vi "asap_monitor.vi"() -> ()   [LabVIEW 2013]
uses:
  <vilib>/Analysis/Matrix/Datatypes/RealMatrix.ctl
  <vilib>/Platform/TimedLoop/XDataNode/timing_clust.ctl
  <vilib>/Platform/TimedLoop/XDataNode/nitl_modes.ctl
  <vilib>/Platform/TimedLoop/XDataNode/wakeup.ctl
  calibration/array_3d_double.ctl
  initialization/micron_globals.vi
  <vilib>/Platform/TimedLoop/XDataNode/XDataNode.xnode
  <vilib>/Platform/TimedLoop/XDataNode/XDNodeRunTimeDep.lvlib
  <vilib>/Analysis/Matrix/NI_Matrix.lvlib
panel:
  in  "To Trace Data":bool
  in  "stop":bool
  in  "Clear":bool
  out "Vector sum":dbl format="%#_4p"
  in  "Display":T1(ring)
  in  "Select":bool[](array[boolean])
  out "ASAP status":cluster{"Valid position":bool, "Message":string}
  out "Match error":sgl[](array[numeric]) format="%#.1f"
  out "Light triad error":dbl[](array[numeric]) format="%#.0f"
  out "Handle pose string":string
  out "Light position":sgl[](array[numeric]) format="%#.0f"
  out "Translation":dbl[](array[numeric]) format="%#.1f"
  out "Sum amplitudes":sgl[][](array[numeric]) format="%#.4f"
  out "Axis position":sgl[](array[numeric]) format="%#_4g"
  out "Total angle":dbl format="%#_4g"
  out "Relative angles":dbl[](array[numeric]) format="%#.1f"
  out "Ref pose":T2=[[1.0, 0.0, 0.0, 0.0], [0.0, 1.0, 0.0, 0.0], [0.0, 0.0, 1.0, 0.0], [0.0, 0.0, 0.0, 1.0]] format="%#.3f"
  in  "Absolute":bool
  out "Sensor views":cluster{sgl[], sgl[]}[](graph)
  in  "Demodulated signals bandwidth":sgl=3.0
  out "Handle pose":T2 format="%#.3f"
  in  "Light":i32
  out "Reference":dbl[][](array[numeric])
  in  "Set ref":bool
  out "Waveform Chart":dbl[][](graph)
  out "Signals":dbl[](array[numeric]) format="%#_4p"
  # "X"
  # "Z1"
  # "Y"
  # "Z2"
  # "Light"
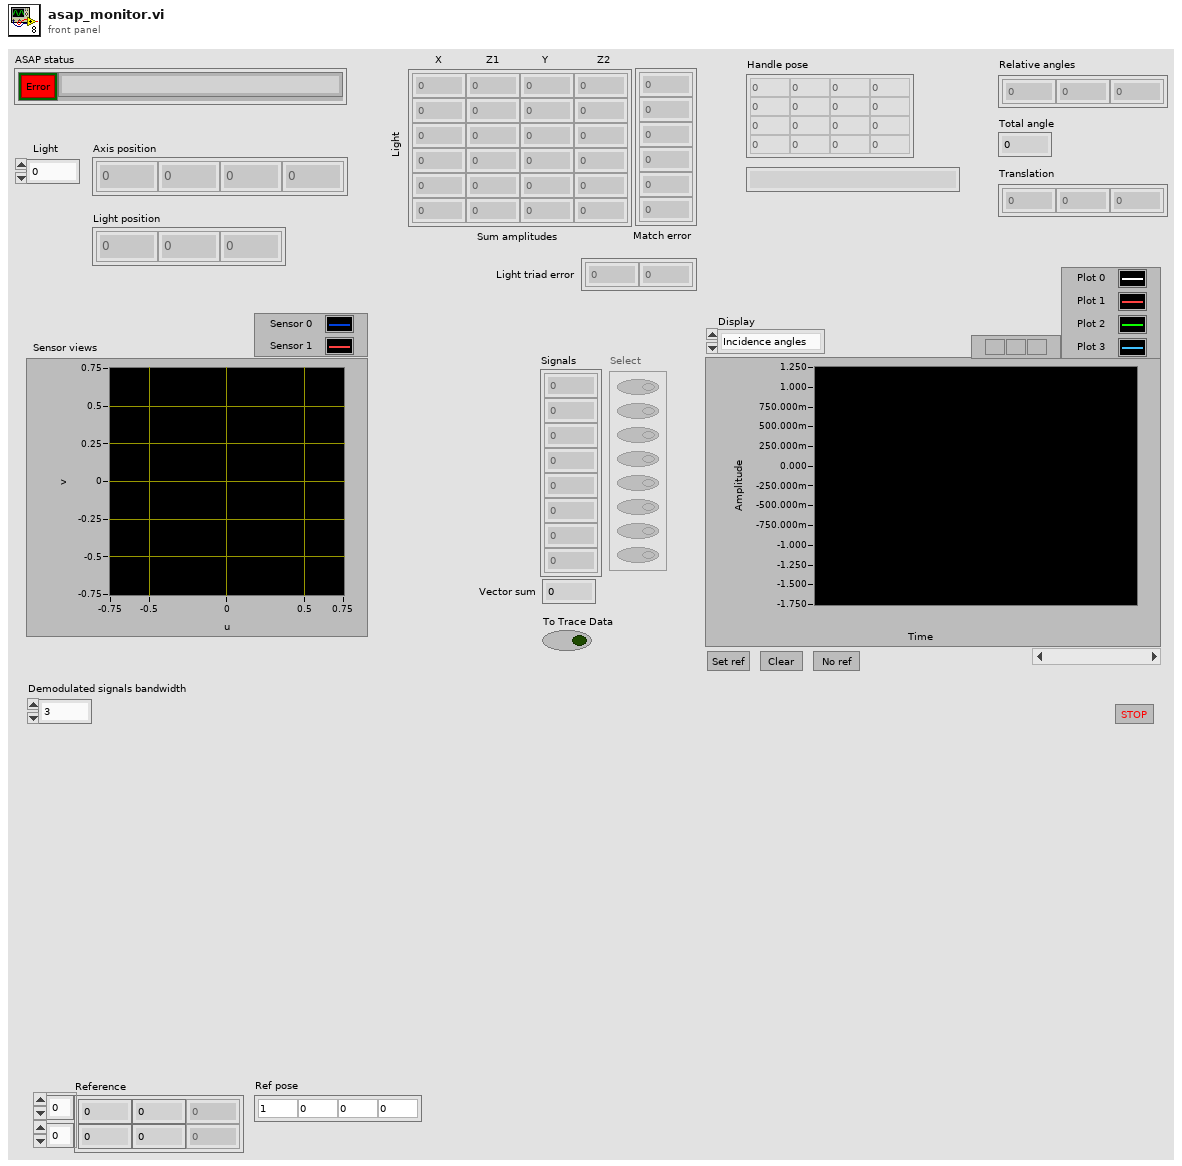
[diagram p1: front panel]
types:
  T1 = enum16{"Incidence angles", "Demod signals", "Sum amplitudes", "Difference signals", "Axis positions", "Light positions"}
  T2 = typedef "NI_Matrix.lvlib/RealMatrix.ctl" = dbl[][]
  T3 = typedef "configuration.ctl" = cluster{"Calibration data":T4, "Block size":i32, "Tasks":cluster{"Analog Input":refnum<k21>, "Counters":refnum<k21>[], "Digital out":refnum<k21>}, "Light enables":bool[]}
  T4 = typedef "asap_calibration.ctl" = cluster{"T1":T2, "K1":T2, "T2":T2, "K2":T2, "Sensor LUT":sgl[][][][]}
  T5 = typedef "micron_config.ctl" = cluster{"rt fifo":refnum<k33>, "Analog output task":refnum<k21>, "Analog output task 2":refnum<k21>, "Stimulus AO task":refnum<k21>, "Low-rate AIN task":refnum<k21>, "Pedal out task":refnum<k21>, "Pedal in task":refnum<k21>, "Loop timing source":string, "Relay out task":refnum<k21>, "Send UDP Conn":refnum<k16>, "Recv UDP Conn":refnum<k16>, "Host Addr":dbl, "I2C interface":T6, "trace_start notifier":refnum<notifier>, "trace_done notifier":refnum<notifier>, "ASAP FIFO":refnum<k33>}
  T6 = typedef "i2c_interface.ctl" = cluster{"FPGA VI Reference":T7}
  T7 = typedef "fpga_reference.ctl" = refnum<k20>
  T8 = typedef "XDNodeRunTimeDep.lvlib/timing_clust.ctl" = cluster{"Expected End [f-1]":u64, "Actual End [f-1]":u64, "Finished Late? [f-1]":bool, "Expected End [i-1]":u64, "Actual End [i-1]":u64, "Finished Late? [i-1]":bool, "Expected Start [i]":u64, "Actual Start [i]":u64, "Expected Start [f]":u64, "Actual Start [f]":u64, "Source Name":string, "Structure Name":string, "Period":i64, "Deadline":i64, "Offset":i64, "Start":i64, "Priority":i32, "Timeout":i32, "Mode":T9, "Wakeup Reason":T10, "Error":errorcluster, "Source Type":string, "Secondary Source Type":string, "Global End Time":u64, "Global Start Time":u64, "Frame Duration":u64, "Iteration Duration":u64, "Assigned CPU":i32, "I/O Scan Engine Mode":u32}
  T9 = typedef "XDNodeRunTimeDep.lvlib/nitl_modes.ctl" = enum32{"No Change", "Process missed periods, maintain original phase", "Discard missed periods, maintain original phase", "Process missed periods, ignore original phase", "Discard missed periods, ignore original phase"}
  T10 = typedef "XDNodeRunTimeDep.lvlib/wakeup.ctl" = enum32{"Normal", "Aborted", "Asynchronous wakeup", "Timing source error", "Timed loop error", "Timeout"}
  T11 = typedef "log_event.ctl" = cluster{"Facility ID":i32, "Severity":enum16{"OK", "Debug", "Warn", "Error"}, "Timestamp":timestamp, "Facility":string, "State":string, "Message":string}
  T12 = cluster{"Axis positions":sgl[], "Axis positions":sgl[]}
  T13 = cluster{"Axis positions":sgl[], "Axis positions":sgl[]}[]
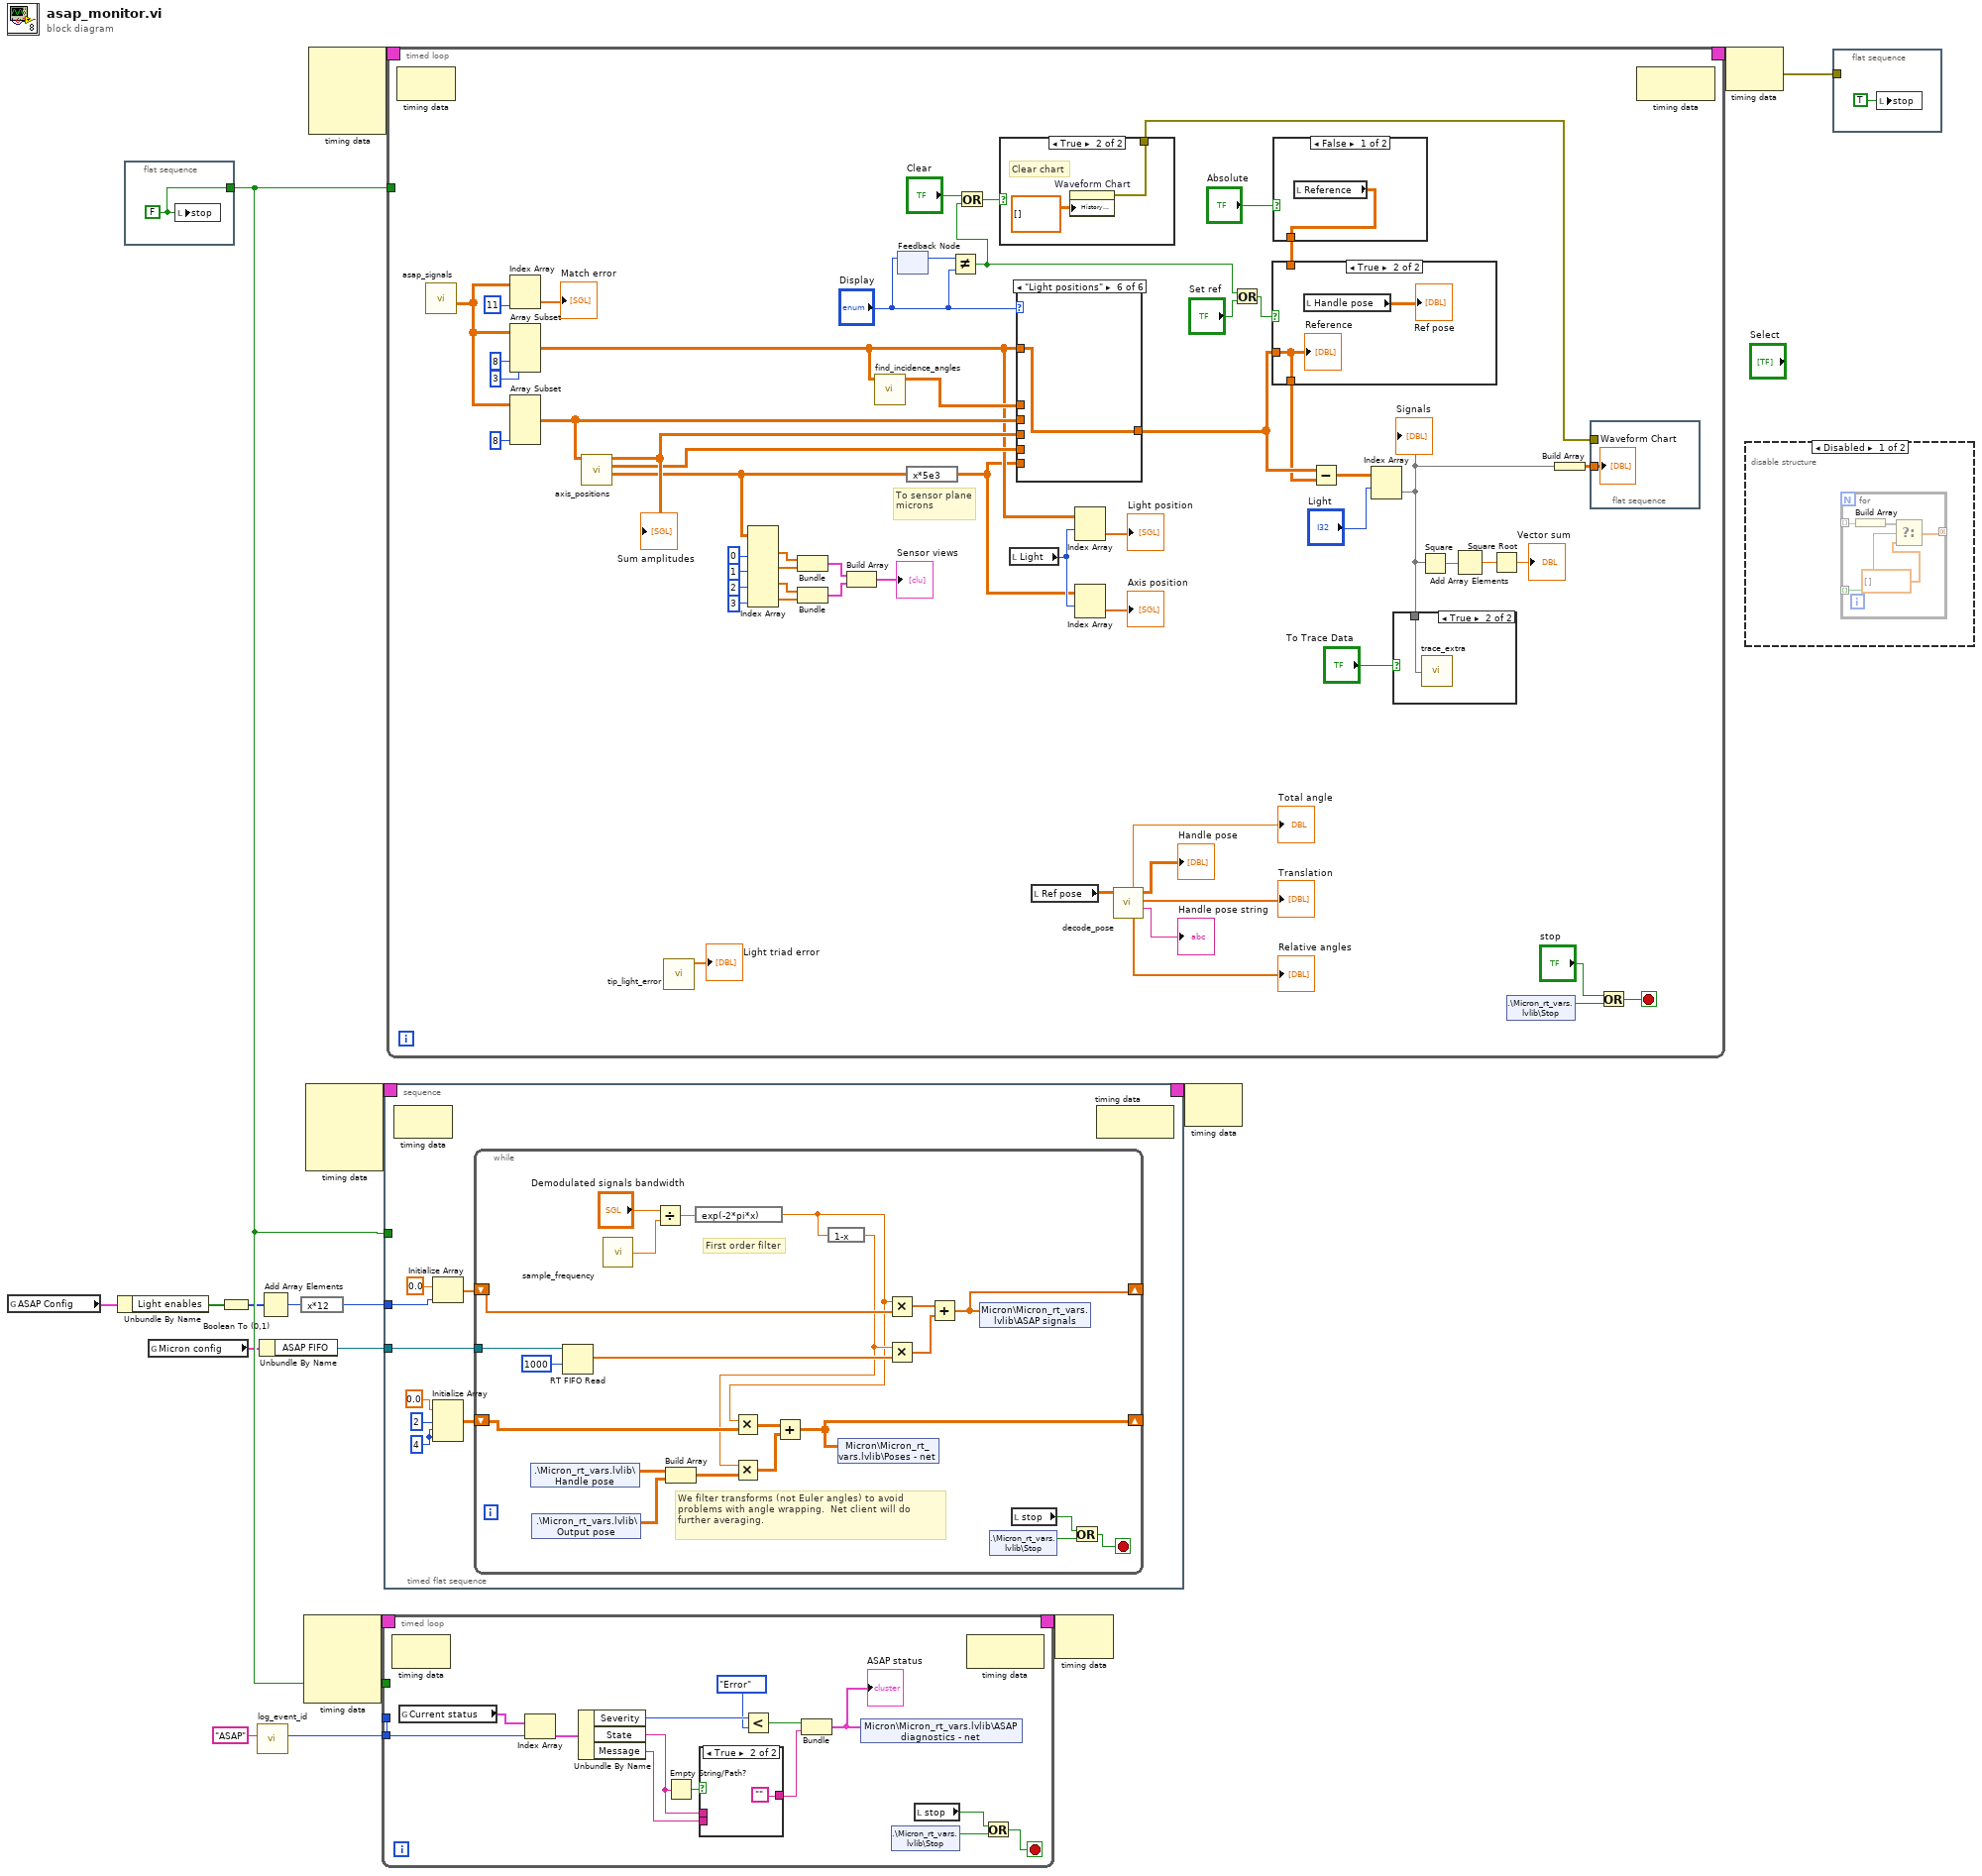
[diagram p0: block diagram]
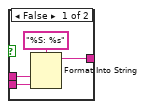
[diagram p3: hidden frame]
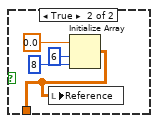
[diagram p11: hidden frame]
diagram:
  n1 = global read "micron_globals.vi" "ASAP Config"() -> (w8:T3)
  n2 = Unbundle By Name(w8) -> ("Light enables"=w9:bool[])
  n3 = flat-sequence {
    tunnel: [w18] -> w17
    frame #0 {
      w18 = FALSE ("stop")
      n4 = local write "stop"(w18) -> ()
    }
  }
  n5 = global read "micron_globals.vi" "Micron config"() -> (w12:T5)
  n6 = Boolean To (0,1)(Boolean=w9) -> (0, 1=w10:i16[])
  n7 = call "log_event_id.vi"("Facility"="ASAP") -> ("Facility ID"=w2:i32)  [unwired: 10 in]
  n8 = Unbundle By Name(w12) -> ("ASAP FIFO"=w11:refnum<k33>)
  n9 = Add Array Elements(numeric array=w10) -> (sum=w7:i16)
  n10 = expression code="x*12"(w7) -> (w6:i16)
  n11 = node-c288() -> (w5:T8)  [unwired: 4 in]
  n12 = node-c288() -> (w14:T8)  [unwired: 4 in]
  n13 = node-c288() -> (w16:T8)  [unwired: 4 in]
  n14 = timed-loop {
    timing: w5 -> [_]
    timing-out: [_] -> w4
    tunnel: [w31] -> _
    tunnel: w2 -> [w31]
    tunnel: w17 -> [_]
    stop <- w19 stop-if-true
    n15 = node-c288() -> ()  [unwired: 1 in, 1 out]
    n16 = global read "micron_globals.vi" "Current status"() -> (w32:T11[])
    n17 = Index Array(array=w32, index=w31) -> (element=w28:T11)
    n18 = Unbundle By Name(w28) -> ("Severity"=w30:enum16{"OK", "Debug", "Warn", "Error"}, "State"=w22:string, "Message"=w25:string)
    n19 = Empty String/Path?(string/path=w22) -> (empty?=w23:bool)
    n20 = case shown="True" w23 {
      tunnel: w22 -> [w35 _]
      tunnel: w25 -> [w34 _]
      tunnel: [w33 ""] -> w24
      frame False {
        n21 = Format Into String(format string="%S: %s", w35, w34) -> (resulting string=w33:string)  [unwired: 2 in, 1 out]
      }
      frame True {
      }
    }
    n22 = Less?(x=w30, y=enum16{"OK", "Debug", "Warn", "Error"}."Error" ("Severity")) -> (x < y?=w27:bool)
    n23 = Bundle(w27, w24) -> (w26:cluster{bool, string})  [unwired: 1 in]
    "ASAP status" <- w26
    n24 = shared-variable "Micron\\Micron_rt_vars.lvlib\\ASAP diagnostics - net"(w26) -> ()  [unwired: 1 in, 1 out]
    n25 = shared-variable ".\\Micron_rt_vars.lvlib\\Stop"() -> (w20:bool)  [unwired: 1 in, 1 out]
    n26 = local read "stop"() -> (w21:bool)
    n27 = node-c288() -> ()  [unwired: 1 in, 1 out]
    n28 = Or(x=w21, y=w20) -> (x .or. y?=w19:bool)
  }
  n29 = timed-sequence {
    timing: w14 -> [_]
    timing-out: [_] -> w13
    tunnel: w11 -> [w42]
    tunnel: w6 -> [w41]
    tunnel: w17 -> [w40]
    n30 = timed-flat-sequence {
      tunnel: w42 -> [w50]
      tunnel: w41 -> [w47]
      tunnel: w40 -> [_]
      w43 = 4 ("dimension size")
      n31 = node-c288() -> ()  [unwired: 1 in, 1 out]
      n32 = Initialize Array(0.0 ("element"), w47) -> (w49:dbl[])
      n33 = Initialize Array(0.0 ("element"), 2 ("dimension size"), w43, w43) -> (w46:dbl[][][])
      n34 = while {
        tunnel: w50 -> [w71]
        shift-right: [w64] -> _
        shift-left: w49 -> [w63]
        shift-right: [w51] -> _
        shift-left: w46 -> [w60]
        stop <- w56 stop-if-true
        # "We filter transforms (not Euler angles) to avoid problems with angle wrapping.  Net client will do further averaging."
        # "First order filter"
        n35 = shared-variable ".\\Micron_rt_vars.lvlib\\Handle pose"() -> (w55:sgl[][])  [unwired: 1 in, 1 out]
        n36 = shared-variable ".\\Micron_rt_vars.lvlib\\Output pose"() -> (w54:sgl[][])  [unwired: 1 in, 1 out]
        n37 = RT FIFO Read(0:w71, 2:1000 ("timeout in ms (0)")) -> (9:w70:sgl[])  [unwired: 2 in, 4 out]
        n38 = call "sample_frequency.vi"() -> ("Sample frequency"=w67:dbl)
        n39 = Divide(x="Demodulated signals bandwidth", y=w67) -> (x/y=w65:dbl)
        n40 = Build Array(w55, w54) -> (w59:sgl[][][])
        n41 = expression code="exp(-2*pi*x)"(w65) -> (w52:dbl)
        n42 = Multiply(x=w52, y=w60) -> (x*y=w61:dbl[][][])
        n43 = expression code="1-x"(w52) -> (w53:dbl)
        n44 = Multiply(x=w53, y=w59) -> (x*y=w62:dbl[][][])
        n45 = Add(x=w61, y=w62) -> (x+y=w51:dbl[][][])
        n46 = shared-variable "Micron\\Micron_rt_vars.lvlib\\Poses - net"(w51) -> ()  [unwired: 1 in, 1 out]
        n47 = Multiply(x=w52, y=w63) -> (x*y=w69:dbl[])
        n48 = Multiply(x=w53, y=w70) -> (x*y=w68:dbl[])
        n49 = Add(x=w69, y=w68) -> (x+y=w64:dbl[])
        n50 = shared-variable "Micron\\Micron_rt_vars.lvlib\\ASAP signals"(w64) -> ()  [unwired: 1 in, 1 out]
        n51 = shared-variable ".\\Micron_rt_vars.lvlib\\Stop"() -> (w58:bool)  [unwired: 1 in, 1 out]
        n52 = local read "stop"() -> (w57:bool)
        n53 = Or(x=w57, y=w58) -> (x .or. y?=w56:bool)
      }
      n54 = node-c288() -> ()  [unwired: 1 in, 1 out]
    }
  }
  n55 = timed-loop {
    timing: w16 -> [_]
    timing-out: [_] -> w15
    tunnel: w17 -> [_]
    stop <- w77 stop-if-true
    # "To sensor plane microns"
    n56 = node-c288() -> ()  [unwired: 1 in, 1 out]
    n57 = call "asap_signals.vi"() -> ("ASAP signals"=w114:sgl[][])  [unwired: 10 in, 1 out]
    n58 = Index Array(array=w114, index (col)=11 ("disabled index (col)")) -> (element=→"Match error":sgl[])  [unwired: 1 in]
    n59 = Array Subset(array=w114, index (col)=8 ("length"), length (col)=3 ("length")) -> (w96:sgl[][])  [unwired: 2 in]
    n60 = Array Subset(array=w114, length (col)=8 ("length")) -> (w98:sgl[][])  [unwired: 3 in]
    n61 = call "axis_positions.vi"("Demodulated signals"=w98) -> ("Axis positions"=w81:sgl[][], "Differences"=w99:sgl[][], "Sum amplitudes"=w100:sgl[][])  [unwired: 8 in]
    "Sum amplitudes" <- w100
    n62 = call "tip_light_error.vi"() -> ("RMS error"=→"Light triad error":dbl[])  [unwired: 11 out]
    n63 = Index Array(array=w81, index (col) #1=0 ("disabled index (col)"), index (col) #2=1 ("index (col)"), index (col) #3=2 ("index (col)"), index (col) #4=3 ("index (col)")) -> (element #1=w127:sgl[], element #2=w126:sgl[], element #3=w125:sgl[], element #4=w124:sgl[])  [unwired: 4 in]
    n64 = Bundle("Axis positions"=w127, "Axis positions"=w126) -> (w123:T12)  [unwired: 1 in]
    n65 = Bundle("Axis positions"=w125, "Axis positions"=w124) -> (w122:T12)  [unwired: 1 in]
    n66 = Build Array(w123, w122) -> (→"Sensor views":T13)
    n67 = call "find_incidence_angles.vi"("Light positions"=w96) -> ("Incidence angles"=w101:dbl[][])  [unwired: 10 in]
    n68 = feedback-in #1("Display") -> ()
    n69 = feedback #1() -> (w95:T1)  [unwired: 1 in]
    n70 = expression code="x*5e3"(w81) -> (w80:sgl[][])
    n71 = Not Equal?(x=w95, y="Display") -> (x != y?=w84:bool)
    n72 = Or(x="Clear", y=w84) -> (x .or. y?=w85:bool)
    n73 = case shown="True" w85 {
      tunnel: [_ w135] -> w93
      frame False {
      }
      frame True {
        # "Clear chart"
        n74 = property on="Waveform Chart" class="WFChart (strict)"("History Data"=dbl[][] []) -> (error out=w135:errorcluster)  [unwired: 2 in, 1 out]
      }
    }
    n75 = local read "Light"() -> (w110:i32)
    n76 = case shown="\"Light positions\"" "Display" {
      tunnel: w101 -> [w136 _ _ _ _ _]
      tunnel: w100 -> [_ _ w138 _ _ _]
      tunnel: w99 -> [_ _ _ w139 _ _]
      tunnel: w98 -> [_ w137 _ _ _ _]
      tunnel: [w136 w137 w138 w139 w140 w141] -> w97
      tunnel: w80 -> [_ _ _ _ w140 _]
      tunnel: w96 -> [_ _ _ _ _ w141]
      frame "Incidence angles", Default {
      }
      frame "Demod signals" {
      }
      frame "Sum amplitudes" {
      }
      frame "Difference signals" {
      }
      frame "Axis positions" {
      }
      frame "Light positions" {
      }
    }
    n77 = local read "Ref pose"() -> (w120:T2)
    n78 = Index Array(array=w96, index (row)=w110) -> (element=→"Light position":sgl[])  [unwired: 1 in]
    n79 = Index Array(array=w80, index (row)=w110) -> (element=→"Axis position":sgl[])  [unwired: 1 in]
    n80 = call "decode_pose.vi"("Ref pose"=w120) -> ("Handle pose string"=→"Handle pose string":string, "Translation"=→"Translation":dbl[], "Handle pose"=→"Handle pose":T2, "Relative angles"=→"Relative angles":dbl[], "Total angle"=→"Total angle":dbl)  [unwired: 6 in]
    n81 = Or(x=w84, y="Set ref") -> (x .or. y?=w90:bool)
    n82 = case shown="False" "Absolute" {
      tunnel: [w142 w143] -> w89
      frame False {
        n83 = local read "Reference"() -> (w142:dbl[][])
      }
      frame True {
        n84 = Initialize Array(0.0 ("X * Y"), 6 ("dimension size"), 8 ("dimension size")) -> (w143:dbl[][])
        n85 = local write "Reference"(w143) -> ()
      }
    }
    n86 = case shown="True" w90 {
      tunnel: w97 -> [_ w148]
      tunnel: w89 -> [w147 _]
      tunnel: [w147 w148] -> w88
      frame False {
      }
      frame True {
        n87 = local read "Handle pose"() -> (→"Ref pose":T2)
        "Reference" <- w148
      }
    }
    n88 = Subtract(x=w97, y=w88) -> (x-y=w104:dbl[][])
    n89 = Index Array(array=w104, index (row)="Light") -> (element=w75:dbl[])  [unwired: 1 in]
    "Signals" <- w75
    n90 = case shown="True" "To Trace Data" {
      tunnel: w75 -> [_ w132]
      frame False {
      }
      frame True {
        n91 = call "trace_extra.vi"("Extra trace data"=w132) -> ()  [unwired: 1 in]
      }
    }
    n92 = Square(x=w75) -> (x^2=w87:dbl[])
    n93 = Add Array Elements(numeric array=w87) -> (sum=w82:dbl)
    n94 = Square Root(x=w82) -> (sqrt(x)=→"Vector sum":dbl)
    n95 = shared-variable ".\\Micron_rt_vars.lvlib\\Stop"() -> (w78:bool)  [unwired: 1 in, 1 out]
    n96 = Build Array(w75) -> (w102:dbl[][])
    n97 = flat-sequence {
      tunnel: w102 -> [w133]
      tunnel: w93 -> [_]
      frame #0 {
        "Waveform Chart" <- w133
      }
    }
    n98 = Or(x="stop", y=w78) -> (x .or. y?=w77:bool)
    n99 = node-c288() -> ()  [unwired: 1 in, 1 out]
  }
  n100 = node-c288(w4) -> ()  [unwired: 1 out]
  n101 = node-c288(w13) -> ()  [unwired: 1 out]
  n102 = node-c288(w15) -> (w1:errorcluster)
  n103 = disable-structure shown="Disabled" {
    frame Disabled {
      n104 = for {
        tunnel: _ -> [w154] mode=indexing
        tunnel: [w156] -> w152 mode=indexing
        tunnel: [w157] -> _ mode=concatenating
        n105 = Build Array(w154) -> (w155:void[])
        n106 = Select(t=w155, s=w156, f=dbl[] []) -> (s? t:f=w157:dbl[])
      }
    }
    frame Enabled {
    }
  }
  n107 = flat-sequence {
    tunnel: w1 -> [_]
    frame #0 {
      n108 = local write "stop"(TRUE ("stop")) -> ()
    }
  }
